vi "Update.vi"(11 "服务器信息":T1={"host"="27.154.58.30", "user"="fb", "password"="std23506", "远端地址"="/725测试平台"}) -> ()   [LabVIEW 2016, in "update.lvlib"]
uses:
  update.lvlib
panel:
  out "滑动杆":dbl(slide) scale=0.0..100.0
  in  "取消按钮":bool
  out "last status string":string caption="最近状态字符串"
  out "command":string caption="命令"
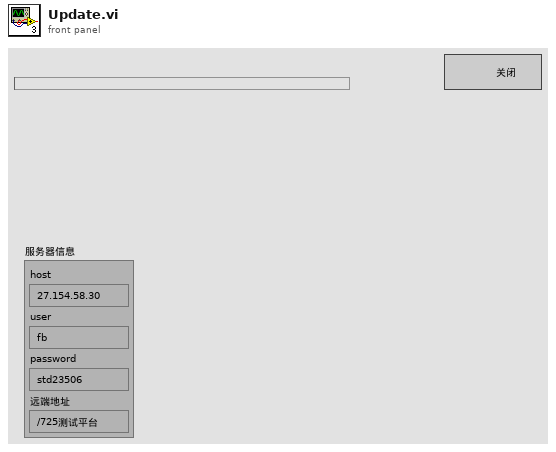
[diagram p1: front panel]
types:
  T1 = cluster{"host":string, "user":string, "password":string, "远端地址":string}
  T2 = cluster{"command":string, "last status string":string, "process":dbl}
  T3 = enum32{"Bad", "Idle", "Run top level", "Running"}
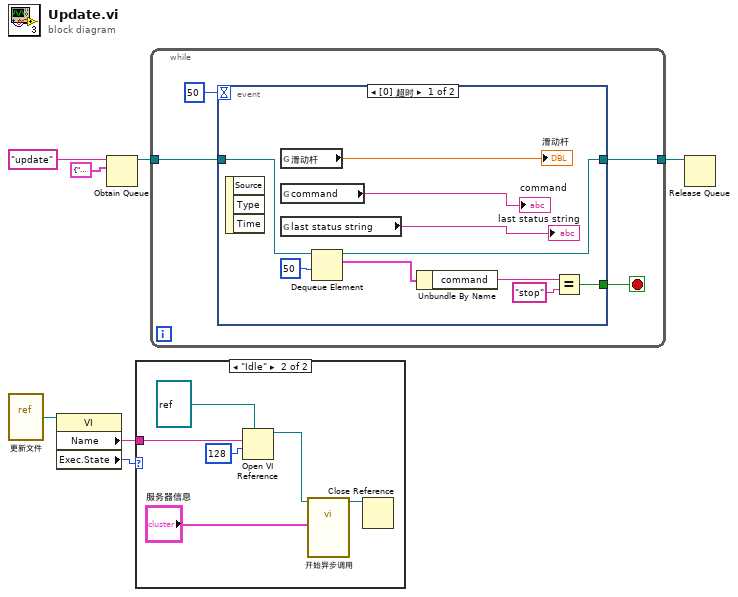
[diagram p0: block diagram]
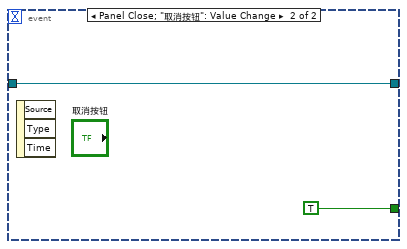
[diagram p3: hidden frame]
diagram:
  n1 = vi-ref "更新文件.vi"() -> (w4:refnum<vi>)
  n2 = property class="VI"(reference=w4) -> ("Name"=w3:string, "Exec.State"=w2:T3)  [unwired: 1 in, 2 out]
  n3 = Obtain Queue(name (unnamed)="update" ("名称（未命名）"), element data type=T2 {"command"="", "last status string"="", "process"=0.0}) -> (queue out=w6:refnum<queue>)  [unwired: 3 in, 2 out]
  n4 = case shown="\"Idle\"" w2 {
    tunnel: w3 -> [_ w13]
    frame "Bad", Default {
    }
    frame "Idle" {
      n5 = Open VI Reference(type specifier VI Refnum (for type only)=refnum<vi> refnum, vi path=w13, options=128 ("选项")) -> (vi reference=w10:refnum<vi>)  [unwired: 3 in, 1 out]
      n6 = call-by-ref "开始异步调用"(reference=w10, "服务器信息"="服务器信息") -> (reference out=w11:refnum<vi>)  [unwired: 12 in, 1 out]
      n7 = Close Reference(reference=w11) -> ()  [unwired: 1 in, 1 out]
    }
  }
  n8 = while {
    tunnel: w6 -> [w15]
    tunnel: [w14] -> w5
    stop <- w16 stop-if-true
    n9 = event shown="[0] 超时" {
      selector: _ -> [_ _]
      dyn-events: _ -> [_ _]
      timeout: 50 -> [_ _]
      tunnel: [w22 TRUE] -> w16
      tunnel: w15 -> [w27 w28]
      tunnel: [w25 w28] -> w14
      event Timeout {
        n10 = event-data() -> ()  [unwired: 1 in, 3 out]
        n11 = global read "更新全局变量.vi" "滑动杆"() -> (→"滑动杆":dbl)
        n12 = global read "更新全局变量.vi" "command"() -> (→"command":string)
        n13 = global read "更新全局变量.vi" "last status string"() -> (→"last status string":string)
        n14 = Dequeue Element(queue=w27, timeout in ms (-1)=50 ("超时毫秒(-1)")) -> (queue out=w25:refnum<queue>, element=w26:T2)  [unwired: 1 in, 2 out]
        n15 = Unbundle By Name(w26) -> ("command"=w24:string)
        n16 = Equal?(x=w24, y="stop") -> (x = y?=w22:bool)
      }
      event Panel Close; "取消按钮": Value Change {
        n17 = event-data() -> ()  [unwired: 1 in, 3 out]
      }
    }
  }
  n18 = Release Queue(queue=w5) -> ()  [unwired: 2 in, 3 out]
